vi "Test Write Complex Number To Serial.vi"() -> ()   [LabVIEW 2014]
uses:
  <vilib>/Aledyne-TSXperts/Arduino Compatible Compiler for LabVIEW/addons/Complex Numbers/Complex Numbers.lvlib
panel:
  out "String complex num.":string
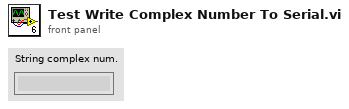
[diagram p1: front panel]
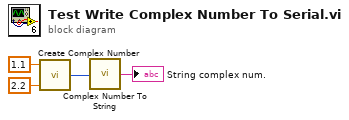
[diagram p0: block diagram]
diagram:
  n1 = call <vilib>:"Create Complex Number.vi"("Imag"=2.2, "Real"=1.1) -> ("Complex"=w4:u32)  [unwired: 3 in]
  n2 = call <vilib>:"Complex Number To String.vi"("Complex number"=w4) -> ("String complex num."=→"String complex num.":string)
